vi "PH_Sequencer.ProcState.vi"(0 "i ref in":refnum<vi>, 2 "state timeout":i32=-1, 4 "state":string, 5 "error in (no error)":errorcluster) -> (14 "i ref out":refnum<vi>, 18 "next state":string, 19 "error out":errorcluster)   [LabVIEW 2014, in "PH_Sequencer.lvlib"]
doc: "This VI represents part of the internal state machine of the object. All methods that are needed to implement the required functionality of the state machine will be called from THIS VI. Add your code here."
uses:
  PH_Sequencer.lvlib
  PH_Beamline/PH_Beamline.Powermeter Instances.ctl
  Z6_Beamline/Z6_Beamline.Powermeter Instances.ctl
  PH_Basics/PH_PP_Common/PH_PP_Common.PUs.ctl
  CS_Core/CSSystem/CoreDefs/CoreDefs.error_type.ctl
  CS_Core/CSSystem/CoreLib/CoreLib.lvlib
  CS_Core/BaseSM/BaseSM.lvlib
  CS_Core/CSSystem/CSSystemLib/CSSystemLib.lvlib
  PH_Classes/PH_Calorimeter_USB/PH_Calorimeter_USB.lvlib
  PH_BackreflectionMeas/PH_BackreflectionMeas.lvlib
  PH_Basics/PH_Common/PH_Common.lvlib
  PH_Beamline/PH_Beamline.lvlib
  PH_Devices/PH_gentec_Powermeter/PH_gentec_Powermeter.lvlib
  Z6_Beamline/Z6_Beamline.lvlib
  PH_Devices/PH_Beckhoff_PPMA-Rods/PH_Beckhoff_PPMA-Rods.lvlib
  PH_BeamlineInformation/PH_BeamlineInformation.lvlib
  PH_Basics/PH_PP_Common/PH_PP_Common.lvlib
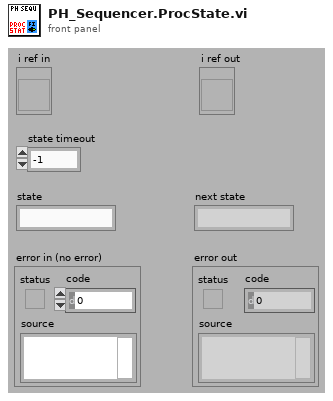
[diagram p1: front panel]
types:
  T1 = typedef "Z6_Beamline.lvlib/Z6_Beamline.Powermeter Instances.ctl" = string
  T2 = typedef "PH_Beamline.lvlib/PH_Beamline.Powermeter Instances.ctl" = string
  T3 = typedef "CoreDefs.error_type.ctl" = enum16{"no error", "can't load process", "can't unload process", "process does not exist", "can't install process", "can't remove process", "unknown function", "time out", "can't execute function", "duplicate queue name", "super not found", "caller queue invalid", "can't ping process", "unknown error", "VISA Error", "VISA timeout", "GPIB timeout", "GPIB error", "communication error", "data type mismatch", "can't read data from OPC server", "can't write data to OPC server", "OET error", "function not implemented", "process already exists", "invalid Shared Variable name", "error writing Shared Variable", "error reading Shared Variable", "invalid client name", "corrupt database", "unknown class", "call not authorized", "parameter out of range", "OET timeout: can't get data to modify", "invalid queue name", "requested operation incompatible with current state", "event undefined", "event disabled", "state undefined", "caller is not a friend", "EventBuilder: bad eventID", "EventBuilder: no DAQ devices", "a thread must not stop itself", "UNUSED ELEMENT4", "DiscArchiver: eventData incomplete", "DiscArchiver: eventData does not belong to run", "DiscArchiver: can't open file", "DiscArchiver: can't write to file", "DiscArchiver: available disc space low", "can't acquire semaphore", "error reading data from database", "notifier object is not existing", "can't register process", "can't unregister process", "illegal event type", "object disabled", "object already exists", "can't change state", "Instrument not found", "no connection to remote node", "invalid reference", "N/A", "UNUSED ELEMENT 1", "element not found", "illegal TCP/IP connection detected", "object does not exist", "invalid access ID", "unknown CS system", "invalid privilige", "unsupported data type", "unsupported server type", "IO server already exists", "Shared Variable already exists"}
  T4 = typedef "PH_Sequencer.lvlib/PH_Sequencer.i attribute.ctl" = cluster{"GUI Refs":cluster{"Main Off":refnum<vi>, "Fire":refnum<vi>, "Status":refnum<vi>, "Ready":refnum<vi>, "Waiting Time":refnum<vi>, "Timeout":refnum<vi>, "PPMA Ready":refnum<vi>, "Sequencer SM State":refnum<vi>, "PPPA Ready":refnum<vi>, "Calorimeter":refnum<vi>, "Beamline Ready":refnum<vi>, "Clear Beamline":refnum<vi>, "Linkage PPMA Rods":refnum<vi>, "Linkage Current PA":refnum<vi>, "Linkage Current MA":refnum<vi>, "Timing Ready":refnum<vi>, "State Timing":refnum<vi>, "Force Timing":refnum<vi>, "PSDB Shot Comment":refnum<vi>, "State PA Backreflection":refnum<vi>, "Beamline Z6 Ready":refnum<vi>, "Clear Z6 Beamline":refnum<vi>, "Sequence length":refnum<vi>, "Timing Mode":refnum<vi>, "Slow Trigger Settings":refnum<vi>, "Experiment Description":refnum<vi>, "State PSDB":refnum<vi>, "PSDB Ready":refnum<vi>, "Set PSDB Settings":refnum<vi>, "Get PSDB Info":refnum<vi>, "Take Snapshot":refnum<vi>, "Shottype":refnum<vi>, "Experiment":refnum<vi>, "Phase Frontends":refnum<vi>, "PP 45mm PILC in use":refnum<vi>}, "Status Info":cluster{"Machine Status":T5, "WaitingTime":i32, "Timeout":bool}, "Readyness":cluster{"Ready to shot":bool, "PPMA Ready":bool, "PPPA Ready":bool, "BL Ready":bool, "Timing Ready":bool, "BL Z6 Ready":bool, "PSDBReady":bool}, "Instancenames":cluster{"PPMA Rods":string, "PP Current Meas":string, "PH Beamline Chief":string, "PA Backrefl Meas":string, "Z6 Beamline Chief":string}, "Data to read":bool, "Calorimeter":cluster{"Instancename":string, "On":bool, "linked":bool}, "Linkage":cluster{"PPMA Rods":bool, "PP Current Meas":bool, "PHELIX Beamline Chief":bool, "PA Backrefl Meas":bool, "Z6 Beamline Chief":bool}, "Timing":cluster{"Instance":string, "linked":bool, "Status":T5, "Timing Mode":T6, "Slow Trigger Settings":T7, "Info available":cluster{"ext SlowTrigger":bool, "T2":bool, "Mode":bool, "Delay Slow Trigger":bool, "Phase FEs":bool}, "FE Phase":T8}, "Service ID R2S":i32, "PSDB":cluster{"Controller Instance":string, "Controller Status":T5, "Controller linked":bool, "Settings acknowledged":bool, "Current Experiment ID":i16, "Current Shot Type":i16, "Current Comment":string, "Remember Settings":bool, "Write 2 early":bool}, "PSDB Data":cluster{"Main Off?":bool, "Sequence Length":dbl, "Sequence startet":timestamp}, "6P 4Q Positions":cluster{"Instancename":string, "linked":bool, "Position":T9}[], "PUs":T10[]}
  T5 = typedef "PH_StatusHandler.lvlib/PH_StatusHandler.Status.ctl" = i16
  T6 = typedef "PH_Timing.lvlib/PH_Timing.Timing Mode.ctl" = cluster{"T2":i16, "Modeselector":enum32{"10 Hz", "0.5 Hz", "Shot"}}
  T7 = typedef "PH_Timing.lvlib/PH_Timing.Slow Trigger Settings.ctl" = cluster{"Delay":dbl, "externally triggered?":bool}
  T8 = typedef "PH_Timing.lvlib/PH_Timing.Phase FEs.ctl" = cluster{"Phase":dbl}
  T9 = typedef "PH_4_Pos_Selector.lvlib/PH_4_Pos_Selector.Position Selector.ctl" = u16
  T10 = typedef "PH_Sequencer.lvlib/PH_Sequencer.Head.ctl" = cluster{"PowerUnit":T11, "GUI Ref":refnum<vi>, "Information":T12, "linked?":bool, "GUI Ref Current Voltage":refnum<vi>}
  T11 = typedef "PH_PP_Common.lvlib/PH_PP_Common.PUs.ctl" = enum16{"no Info", "PA-19mm-1", "PA-19mm-2", "PA-45mm-PILC", "PA-45mm-MAIN", "MA-PU-1", "MA-PU-2", "MA-PU-3", "MA-PU-4", "MA-PU-5", "MA-PU-6", "MA-FR", "MA-PILC", "PA-45mm-DP"}
  T12 = typedef "PH_Sequencer.lvlib/PH_Sequencer.PU Information.ctl" = cluster{"State":T5, "Waiting Time [s]":dbl, "PU State SM":T13, "PU Timeout SM":T13}
  T13 = typedef "PH_PowerUnit_BaseClass.lvlib/PH_PowerUnit_BaseClass.SM States.ctl" = enum16{".", "Stand by", "Switch PU on", "Configure", "Set Default Voltage", "Set STANDBY", "Set READY", "Wait for Shot Cmd", "Open Dump Rods", "Open Ross Relais", "Close Ross Relais", "Switch PSU on", "Switch PSU off", "Charge", "Switch GD Channel on", "Close Dump Rods", "Rods-TO", "RR-TO", "PSU-TO", "Trigger-TO"}
  T14 = typedef "PH_BeamlineInformation.lvlib/PH_BeamlineInformation.i attribute.ctl" = cluster{"BL GUI Elements of Services":cluster{"Service Name":string, "GUI Elements":refnum<vi>[], "Status":i32}[], "Powermeters":T15, "Efficiency":T16, "Heads":T17[]}
  T15 = typedef "PH_BeamlineInformation.lvlib/PH_BeamlineInformation.Powermeter.ctl" = cluster{"ns FE":cluster{"GUI Ref":refnum<vi>, "Value":dbl}, "fs FE":cluster{"GUI Ref":refnum<vi>, "Value":dbl}, "PA":cluster{"GUI Ref":refnum<vi>, "Value":dbl}, "MA":cluster{"GUI Ref":refnum<vi>, "Value":dbl}, "Z6 green":cluster{"GUI Ref":refnum<vi>, "Value":dbl}, "Z6 IR":cluster{"GUI Ref":refnum<vi>, "Value":dbl}, "Z6 COS":cluster{"GUI Ref":refnum<vi>, "Value":dbl}}
  T16 = typedef "PH_BeamlineInformation.lvlib/PH_BeamlineInformation.Efficiency.ctl" = cluster{"PA Gain":cluster{"GUI Ref":refnum<vi>, "Value":dbl}, "MA Gain":cluster{"GUI Ref":refnum<vi>, "Value":dbl}, "Z6 green Conversion":cluster{"GUI Ref":refnum<vi>, "Value":dbl}, "Z6 Comp Losses":cluster{"GUI Ref":refnum<vi>, "Value":dbl}}
  T17 = typedef "PH_BeamlineInformation.lvlib/PH_BeamlineInformation.Head.ctl" = cluster{"PowerUnit":T11, "in use":cluster{"Value":bool, "GUI Ref":refnum<vi>, "linked":bool}, "voltage":cluster{"Value":dbl, "GUI Ref":refnum<vi>, "linked":bool}}
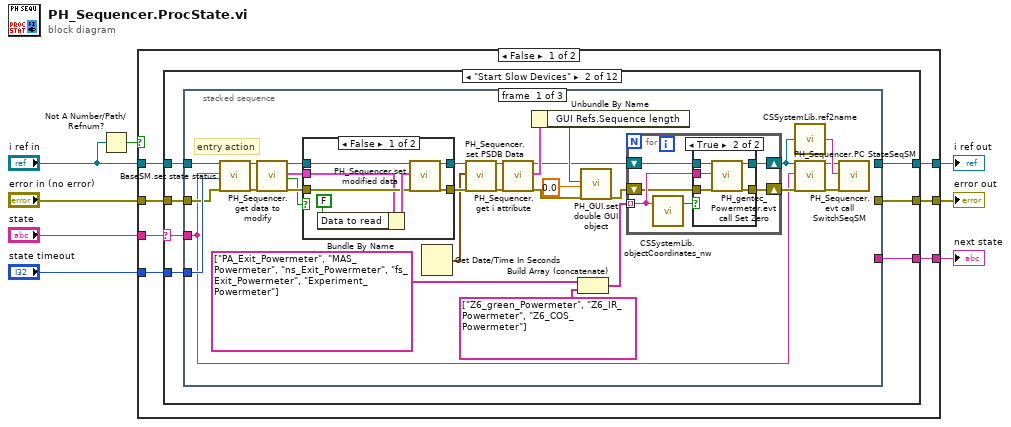
[diagram p0: block diagram]
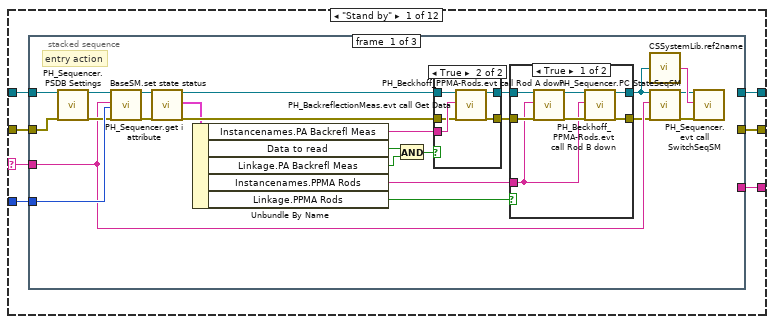
[diagram p2: hidden frame]
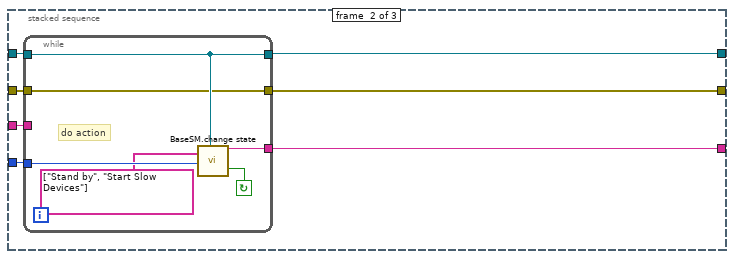
[diagram p5: hidden frame]
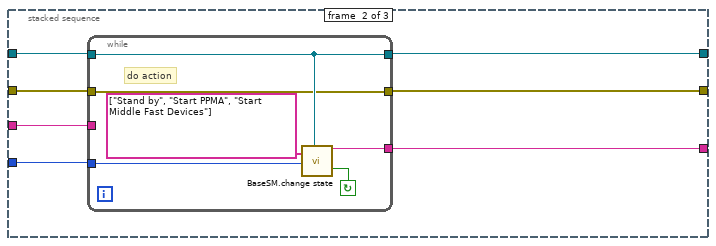
[diagram p9: hidden frame]
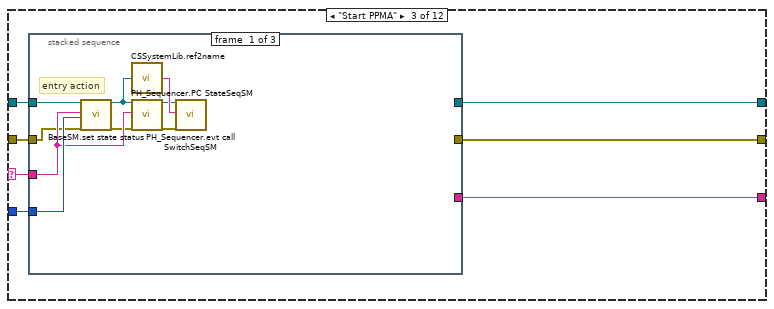
[diagram p11: hidden frame]
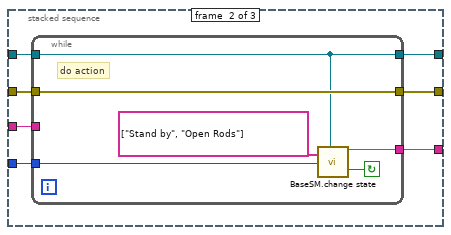
[diagram p12: hidden frame]
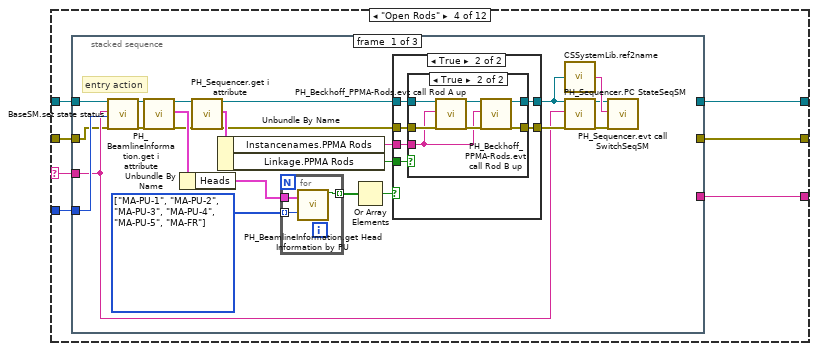
[diagram p14: hidden frame]
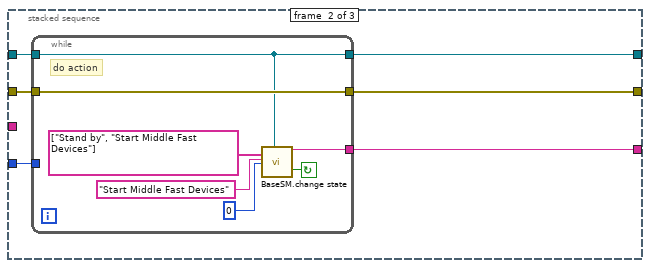
[diagram p17: hidden frame]
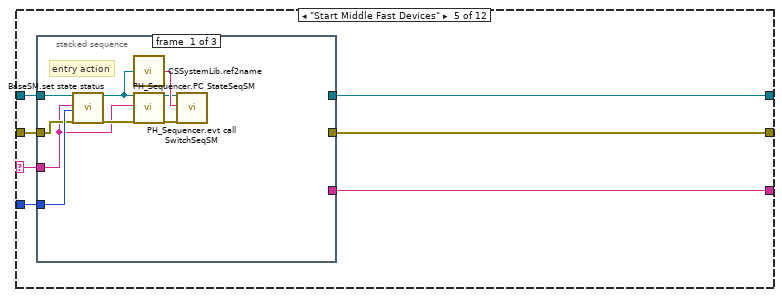
[diagram p19: hidden frame]
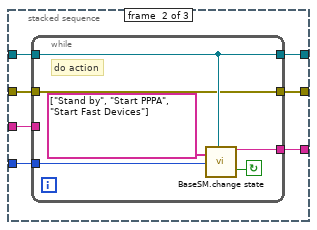
[diagram p20: hidden frame]
diagram:
  n1 = Not A Number/Path/Refnum?(number/path/refnum="i ref in") -> (NaN/Path/Refnum?=w2:bool)
  n2 = case shown="False" w2 {
    tunnel: "i ref in" -> [w15 w474]
    tunnel: [w14 w474] -> w8
    tunnel: "state" -> [w13 w471]
    tunnel: [w12 w471] -> w6
    tunnel: "state timeout" -> [w11 _]
    tunnel: "error in (no error)" -> [w10 _]
    tunnel: [w9 w472] -> w3
    frame False {
      n3 = case shown="\"Start Slow Devices\"" w13 {
        selector: w13 -> [w22 w82 w153 w181 w242 w271 w301 w344 w372 w400 w428 w465]
        tunnel: w15 -> [w20 w80 w151 w179 w240 w269 w299 w342 w370 w398 w426 w470]
        tunnel: [w19 w79 w150 w178 w239 w268 w298 w341 w369 w397 w425 w469] -> w14
        tunnel: [w21 w81 w152 w180 w241 w270 w300 w343 w371 w399 w427 w464] -> w12
        tunnel: w11 -> [w18 w78 w149 w177 w238 w267 w297 w340 w368 w396 w424 w466]
        tunnel: w10 -> [w17 w77 w148 w176 w237 w266 w296 w339 w367 w395 w423 w468]
        tunnel: [w16 w76 w147 w175 w236 w265 w295 w338 w366 w394 w422 w467] -> w9
        frame "Stand by" {
          n4 = stacked-sequence {
            tunnel: w22 -> [w31 w69 _]
            tunnel: [_ w68 _] -> w21
            tunnel: w20 -> [w40 w66 _]
            tunnel: [_ w65 _] -> w19
            tunnel: w18 -> [w39 w67 _]
            tunnel: w17 -> [w42 w63 _]
            tunnel: [_ w64 _] -> w16
            frame #0 {
              # "entry action"
              n5 = call "PH_Sequencer.PSDB Settings.vi"("i ref in"=w40, "error in"=w42) -> ("i ref out"=w38:refnum<vi>, "error out"=w36:errorcluster)  [unwired: 16 in]
              n6 = call "BaseSM.set state status.vi"("i ref in"=w38, "stateStatus"=w31, "ms timeout (10000)"=w39, "error in (no error)"=w36) -> ("i ref out"=w37:refnum<vi>, "error out"=w35:errorcluster)  [unwired: 13 in, 1 out]
              n7 = call "PH_Sequencer.get i attribute.vi"("i ref in"=w37, "error in (no error)"=w35) -> ("i ref out"=w44:refnum<vi>, "i attribute"=w41:T4, "error out"=w43:errorcluster)  [unwired: 15 in]
              n8 = Unbundle By Name(w41) -> ("Instancenames.PA Backrefl Meas"=w23:string, "Data to read"=w25:bool, "Linkage.PA Backrefl Meas"=w24:bool, "Instancenames.PPMA Rods"=w30:string, "Linkage.PPMA Rods"=w29:bool)
              n9 = And(x=w25, y=w24) -> (x .and. y?=w26:bool)
              n10 = case shown="True" w26 {
                tunnel: w44 -> [w48 w49]
                tunnel: [w48 w53] -> w46
                tunnel: w43 -> [w47 w50]
                tunnel: [w47 w52] -> w45
                tunnel: w23 -> [_ w51]
                frame False {
                }
                frame True {
                  n11 = call "PH_BackreflectionMeas.evt call Get Data.vi"("i ref in"=w49, "Instance"=w51, "error in (no error)"=w50) -> ("i ref out"=w53:refnum<vi>, "error out"=w52:errorcluster)  [unwired: 15 in]
                }
              }
              n12 = case shown="True" w29 {
                tunnel: w46 -> [w60 w62]
                tunnel: [w55 w62] -> w28
                tunnel: w45 -> [w59 w61]
                tunnel: [w57 w61] -> w27
                tunnel: w30 -> [w54 _]
                frame True {
                  n13 = call "PH_Beckhoff_PPMA-Rods.evt call Rod A down.vi"("i ref in"=w60, "Instance name"=w54, "error in"=w59) -> ("i ref out"=w56:refnum<vi>, "error out"=w58:errorcluster)  [unwired: 15 in]
                  n14 = call "PH_Beckhoff_PPMA-Rods.evt call Rod B down.vi"("i ref in"=w56, "Instance name"=w54, "error in"=w58) -> ("i ref out"=w55:refnum<vi>, "error out"=w57:errorcluster)  [unwired: 15 in]
                }
                frame False {
                }
              }
              n15 = call "CSSystemLib.ref2name.vi"("obj refnum"=w28) -> ("name"=w34:string)
              n16 = call "PH_Sequencer.PC StateSeqSM.vi"("i ref in"=w28, "Seq SM State"=w31, "error in (no error)"=w27) -> ("i ref out"=w33:refnum<vi>, "error out"=w32:errorcluster)  [unwired: 15 in]
              n17 = call "PH_Sequencer.evt call SwitchSeqSM.vi"("i ref in"=w33, "Instance"=w34, "error in (no error)"=w32) -> ()  [unwired: 15 in, 2 out]
            }
            frame #1 {
              n18 = while {
                tunnel: w67 -> [w73]
                tunnel: [w75] -> w68
                tunnel: w69 -> [_]
                tunnel: w66 -> [w72]
                tunnel: [w72] -> w65
                tunnel: [w71] -> w64
                tunnel: w63 -> [w71]
                stop <- w74 continue-if-true
                # "do action"
                n19 = call "BaseSM.change state.vi"("allowed next states"=string[] ["Stand by", "Start Slow Devices"], "wait time [ms]"=w73, "i ref in"=w72) -> ("next state"=w75:string, "continue loop"=w74:bool)  [unwired: 13 in, 2 out]
              }
            }
            frame #2 {
              # "exit action"
            }
          }
        }
        frame "Start Slow Devices" {
          n20 = stacked-sequence {
            tunnel: w82 -> [w87 w140 _]
            tunnel: [_ w139 _] -> w81
            tunnel: w80 -> [w110 w137 _]
            tunnel: [_ w136 _] -> w79
            tunnel: w78 -> [w111 w138 _]
            tunnel: w77 -> [w109 w134 _]
            tunnel: [_ w135 _] -> w76
            frame #0 {
              # "entry action"
              n21 = call "BaseSM.set state status.vi"("i ref in"=w110, "stateStatus"=w87, "ms timeout (10000)"=w111, "error in (no error)"=w109) -> ("i ref out"=w108:refnum<vi>, "error out"=w106:errorcluster)  [unwired: 13 in, 1 out]
              n22 = call "PH_Sequencer.get data to modify.vi"("i ref in"=w108, "error in (no error)"=w106) -> ("i ref out"=w107:refnum<vi>, "i attribute"=w103:T4, "timed out"=w104:bool, "error out"=w105:errorcluster)  [unwired: 14 in]
              n23 = case shown="False" w104 {
                tunnel: w103 -> [w127 _]
                tunnel: w107 -> [w129 w133]
                tunnel: w105 -> [w128 w132]
                tunnel: [w126 w133] -> w94
                tunnel: [w125 w132] -> w96
                frame False {
                  n24 = Bundle By Name(cluster=w127, "Data to read"=FALSE) -> (w131:T4)
                  n25 = call "PH_Sequencer.set modified data.vi"("i ref in"=w129, "i attribute"=w131, "error in (no error)"=w128) -> ("i ref out"=w126:refnum<vi>, "error out"=w125:errorcluster)  [unwired: 15 in]
                }
                frame True {
                }
              }
              n26 = Get Date/Time In Seconds() -> (seconds since 1Jan1904=w93:timestamp)
              n27 = call "PH_Sequencer.set PSDB Data.vi"("i ref in"=w94, "Start Sequence Time (0)"=w93, "error in"=w96) -> ("i ref out"=w95:refnum<vi>, "error out"=w97:errorcluster)  [unwired: 15 in]
              n28 = call "PH_Sequencer.get i attribute.vi"("i ref in"=w95, "error in (no error)"=w97) -> ("i ref out"=w84:refnum<vi>, "i attribute"=w102:T4, "error out"=w83:errorcluster)  [unwired: 15 in]
              n29 = Unbundle By Name(w102) -> ("GUI Refs.Sequence length"=w101:refnum<vi>)
              n30 = Build Array (concatenate)(T2[] ["PA_Exit_Powermeter", "MAS_Powermeter", "ns_Exit_Powermeter", "fs_Exit_Powermeter", "Experiment_Powermeter"], T1[] ["Z6_green_Powermeter", "Z6_IR_Powermeter", "Z6_COS_Powermeter"]) -> (w98:T1[])
              n31 = call "PH_GUI.set double GUI object.vi"("GUI object Ref"=w101, "value"=0.0, "error in (no error)"=w83) -> ("error out"=w86:errorcluster)  [unwired: 16 in]
              n32 = for {
                tunnel: w98 -> [w117] mode=indexing
                shift-right: [w115] -> w89
                shift-left: w84 -> [w114]
                shift-right: [w113] -> w88
                shift-left: w86 -> [w112]
                n33 = call "CSSystemLib.objectCoordinates_nw.vi"("name"=w117) -> ("obj exists"=w116:bool)  [unwired: 15 in, 3 out]
                n34 = case shown="True" w116 {
                  tunnel: w117 -> [_ w124]
                  tunnel: [w119 w123] -> w115
                  tunnel: w114 -> [w119 w122]
                  tunnel: [w118 w121] -> w113
                  tunnel: w112 -> [w118 w120]
                  frame False {
                  }
                  frame True {
                    n35 = call "PH_gentec_Powermeter.evt call Set Zero.vi"("i ref in"=w122, "Instance"=w124, "error in (no error)"=w120) -> ("i ref out"=w123:refnum<vi>, "error out"=w121:errorcluster)  [unwired: 15 in]
                  }
                }
              }
              n36 = call "CSSystemLib.ref2name.vi"("obj refnum"=w89) -> ("name"=w92:string)
              n37 = call "PH_Sequencer.PC StateSeqSM.vi"("i ref in"=w89, "Seq SM State"=w87, "error in (no error)"=w88) -> ("i ref out"=w91:refnum<vi>, "error out"=w90:errorcluster)  [unwired: 15 in]
              n38 = call "PH_Sequencer.evt call SwitchSeqSM.vi"("i ref in"=w91, "Instance"=w92, "error in (no error)"=w90) -> ()  [unwired: 15 in, 2 out]
            }
            frame #1 {
              n39 = while {
                tunnel: w138 -> [w141]
                tunnel: [w146] -> w139
                tunnel: w140 -> [_]
                tunnel: w137 -> [w144]
                tunnel: [w144] -> w136
                tunnel: [w143] -> w135
                tunnel: w134 -> [w143]
                stop <- w145 continue-if-true
                # "do action"
                n40 = call "BaseSM.change state.vi"("allowed next states"=string[] ["Stand by", "Start PPMA", "Start Middle Fast Devices"], "wait time [ms]"=w141, "i ref in"=w144) -> ("next state"=w146:string, "continue loop"=w145:bool)  [unwired: 13 in, 2 out]
              }
            }
            frame #2 {
              # "exit action"
            }
          }
        }
        frame "Start PPMA" {
          n41 = stacked-sequence {
            tunnel: w153 -> [w158 w168 _]
            tunnel: [_ w167 _] -> w152
            tunnel: w151 -> [w160 w165 _]
            tunnel: [_ w164 _] -> w150
            tunnel: w149 -> [w161 w166 _]
            tunnel: w148 -> [w155 w162 _]
            tunnel: [_ w163 _] -> w147
            frame #0 {
              # "entry action"
              n42 = call "BaseSM.set state status.vi"("i ref in"=w160, "stateStatus"=w158, "ms timeout (10000)"=w161, "error in (no error)"=w155) -> ("i ref out"=w154:refnum<vi>)  [unwired: 13 in, 2 out]
              n43 = call "CSSystemLib.ref2name.vi"("obj refnum"=w154) -> ("name"=w159:string)
              n44 = call "PH_Sequencer.PC StateSeqSM.vi"("i ref in"=w154, "Seq SM State"=w158, "error in (no error)"=w155) -> ("i ref out"=w157:refnum<vi>, "error out"=w156:errorcluster)  [unwired: 15 in]
              n45 = call "PH_Sequencer.evt call SwitchSeqSM.vi"("i ref in"=w157, "Instance"=w159, "error in (no error)"=w156) -> ()  [unwired: 15 in, 2 out]
            }
            frame #1 {
              n46 = while {
                tunnel: w166 -> [w171]
                tunnel: [w174] -> w167
                tunnel: w168 -> [_]
                tunnel: w165 -> [w169]
                tunnel: [w169] -> w164
                tunnel: [w170] -> w163
                tunnel: w162 -> [w170]
                stop <- w173 continue-if-true
                # "do action"
                n47 = call "BaseSM.change state.vi"("allowed next states"=string[] ["Stand by", "Open Rods"], "wait time [ms]"=w171, "i ref in"=w169) -> ("next state"=w174:string, "continue loop"=w173:bool)  [unwired: 13 in, 2 out]
              }
            }
            frame #2 {
              # "exit action"
            }
          }
        }
        frame "Open Rods" {
          n48 = stacked-sequence {
            tunnel: w181 -> [w198 _ _]
            tunnel: [_ w228 _] -> w180
            tunnel: w179 -> [w188 w226 _]
            tunnel: [_ w225 _] -> w178
            tunnel: w177 -> [w202 w227 _]
            tunnel: w176 -> [w186 w223 _]
            tunnel: [_ w224 _] -> w175
            frame #0 {
              w182 = T11[] [enum."MA-PU-1", enum."MA-PU-2", enum."MA-PU-3", enum."MA-PU-4", enum."MA-PU-5", enum."MA-FR"] items=["no Info", "PA-19mm-1", "PA-19mm-2", "PA-45mm-PILC", "PA-45mm-MAIN", "MA-PU-1", "MA-PU-2", "MA-PU-3", "MA-PU-4", "MA-PU-5", "MA-PU-6", "MA-FR", "MA-PILC", "PA-45mm-DP"]
              # "entry action"
              n49 = call "BaseSM.set state status.vi"("i ref in"=w188, "stateStatus"=w198, "ms timeout (10000)"=w202, "error in (no error)"=w186) -> ()  [unwired: 13 in, 3 out]
              n50 = call "PH_BeamlineInformation.get i attribute.vi"("i ref in"=w188, "error in (no error)"=w186) -> ("i ref out"=w187:refnum<vi>, "i attribute"=w189:T14, "error out"=w185:errorcluster)  [unwired: 15 in]
              n51 = Unbundle By Name(w189) -> ("Heads"=w184:T17[])
              n52 = call "PH_Sequencer.get i attribute.vi"("i ref in"=w187, "error in (no error)"=w185) -> ("i ref out"=w193:refnum<vi>, "i attribute"=w197:T4, "error out"=w194:errorcluster)  [unwired: 15 in]
              n53 = Unbundle By Name(w197) -> ("Instancenames.PPMA Rods"=w196:string, "Linkage.PPMA Rods"=w195:bool)
              n54 = for {
                tunnel: [w205] -> w183 mode=indexing
                tunnel: w184 -> [w204]
                tunnel: w182 -> [w203] mode=indexing
                n55 = call "PH_BeamlineInformation.get Head Information by PU.vi"("Heads"=w204, "Power Unit"=w203) -> ("In Use?"=w205:bool)  [unwired: 12 in, 5 out]
              }
              n56 = Or Array Elements(Boolean array=w183) -> (logical OR=w201:bool)
              n57 = case shown="True" w201 {
                tunnel: w193 -> [w207 w213]
                tunnel: [w207 w212] -> w190
                tunnel: w194 -> [w206 w211]
                tunnel: [w206 w210] -> w199
                tunnel: w196 -> [_ w209]
                tunnel: w195 -> [_ w208]
                frame False {
                }
                frame True {
                  n58 = case shown="True" w208 {
                    tunnel: w213 -> [w215 w222]
                    tunnel: [w215 w216] -> w212
                    tunnel: w211 -> [w214 w221]
                    tunnel: [w214 w219] -> w210
                    tunnel: w209 -> [_ w218]
                    frame False {
                    }
                    frame True {
                      n59 = call "PH_Beckhoff_PPMA-Rods.evt call Rod A up.vi"("i ref in"=w222, "Instance name"=w218, "error in"=w221) -> ("i ref out"=w217:refnum<vi>, "error out"=w220:errorcluster)  [unwired: 15 in]
                      n60 = call "PH_Beckhoff_PPMA-Rods.evt call Rod B up.vi"("i ref in"=w217, "Instance name"=w218, "error in"=w220) -> ("i ref out"=w216:refnum<vi>, "error out"=w219:errorcluster)  [unwired: 15 in]
                    }
                  }
                }
              }
              n61 = call "CSSystemLib.ref2name.vi"("obj refnum"=w190) -> ("name"=w200:string)
              n62 = call "PH_Sequencer.PC StateSeqSM.vi"("i ref in"=w190, "Seq SM State"=w198, "error in (no error)"=w199) -> ("i ref out"=w191:refnum<vi>, "error out"=w192:errorcluster)  [unwired: 15 in]
              n63 = call "PH_Sequencer.evt call SwitchSeqSM.vi"("i ref in"=w191, "Instance"=w200, "error in (no error)"=w192) -> ()  [unwired: 15 in, 2 out]
            }
            frame #1 {
              n64 = while {
                tunnel: w227 -> [_]
                tunnel: [w235] -> w228
                tunnel: w226 -> [w229]
                tunnel: [w229] -> w225
                tunnel: [w230] -> w224
                tunnel: w223 -> [w230]
                stop <- w234 continue-if-true
                # "do action"
                n65 = call "BaseSM.change state.vi"("allowed next states"=string[] ["Stand by", "Start Middle Fast Devices"], "default state"="Start Middle Fast Devices", "wait time [ms]"=0 ("wait time"), "i ref in"=w229) -> ("next state"=w235:string, "continue loop"=w234:bool)  [unwired: 12 in, 2 out]
              }
            }
            frame #2 {
              # "exit action"
            }
          }
        }
        frame "Start Middle Fast Devices" {
          n66 = stacked-sequence {
            tunnel: w242 -> [w246 w258 _]
            tunnel: [_ w257 _] -> w241
            tunnel: w240 -> [w250 w255 _]
            tunnel: [_ w254 _] -> w239
            tunnel: w238 -> [w251 w256 _]
            tunnel: w237 -> [w249 w252 _]
            tunnel: [_ w253 _] -> w236
            frame #0 {
              # "entry action"
              n67 = call "BaseSM.set state status.vi"("i ref in"=w250, "stateStatus"=w246, "ms timeout (10000)"=w251, "error in (no error)"=w249) -> ("i ref out"=w244:refnum<vi>, "error out"=w247:errorcluster)  [unwired: 13 in, 1 out]
              n68 = call "CSSystemLib.ref2name.vi"("obj refnum"=w244) -> ("name"=w248:string)
              n69 = call "PH_Sequencer.PC StateSeqSM.vi"("i ref in"=w244, "Seq SM State"=w246, "error in (no error)"=w247) -> ("i ref out"=w243:refnum<vi>, "error out"=w245:errorcluster)  [unwired: 15 in]
              n70 = call "PH_Sequencer.evt call SwitchSeqSM.vi"("i ref in"=w243, "Instance"=w248, "error in (no error)"=w245) -> ()  [unwired: 15 in, 2 out]
            }
            frame #1 {
              n71 = while {
                tunnel: w256 -> [w259]
                tunnel: [w264] -> w257
                tunnel: w258 -> [_]
                tunnel: w255 -> [w262]
                tunnel: [w262] -> w254
                tunnel: [w261] -> w253
                tunnel: w252 -> [w261]
                stop <- w263 continue-if-true
                # "do action"
                n72 = call "BaseSM.change state.vi"("allowed next states"=string[] ["Stand by", "Start PPPA", "Start Fast Devices"], "wait time [ms]"=w259, "i ref in"=w262) -> ("next state"=w264:string, "continue loop"=w263:bool)  [unwired: 13 in, 2 out]
              }
            }
            frame #2 {
              # "exit action"
            }
          }
        }
        frame "Start PPPA" {
          # "To wait for 2.5 s is due to PA 45mm DP:\nWithin this state, the hardware gets ready (takes some time)\nat \"Start Fast Devices\" the charge command is given."
          n73 = stacked-sequence {
            tunnel: w271 -> [w278 w287 _]
            tunnel: [_ w286 _] -> w270
            tunnel: w269 -> [w275 w284 _]
            tunnel: [_ w283 _] -> w268
            tunnel: w267 -> [w280 w285 _]
            tunnel: w266 -> [w274 w281 _]
            tunnel: [_ w282 _] -> w265
            frame #0 {
              # "entry action"
              n74 = call "BaseSM.set state status.vi"("i ref in"=w275, "stateStatus"=w278, "ms timeout (10000)"=w280, "error in (no error)"=w274) -> ("i ref out"=w273:refnum<vi>, "error out"=w272:errorcluster)  [unwired: 13 in, 1 out]
              n75 = call "CSSystemLib.ref2name.vi"("obj refnum"=w273) -> ("name"=w279:string)
              n76 = call "PH_Sequencer.PC StateSeqSM.vi"("i ref in"=w273, "Seq SM State"=w278, "error in (no error)"=w272) -> ("i ref out"=w276:refnum<vi>, "error out"=w277:errorcluster)  [unwired: 15 in]
              n77 = call "PH_Sequencer.evt call SwitchSeqSM.vi"("i ref in"=w276, "Instance"=w279, "error in (no error)"=w277) -> ()  [unwired: 15 in, 2 out]
            }
            frame #1 {
              n78 = while {
                tunnel: w285 -> [_]
                tunnel: [w294] -> w286
                tunnel: w287 -> [_]
                tunnel: w284 -> [w288]
                tunnel: [w288] -> w283
                tunnel: [w289] -> w282
                tunnel: w281 -> [w289]
                stop <- w293 continue-if-true
                # "do action"
                n79 = call "BaseSM.change state.vi"("allowed next states"=string[] ["Stand by", "Start Fast Devices"], "default state"="Start Fast Devices", "wait time [ms]"=2500 ("wait time"), "i ref in"=w288) -> ("next state"=w294:string, "continue loop"=w293:bool)  [unwired: 12 in, 2 out]
              }
            }
            frame #2 {
              # "exit action"
            }
          }
        }
        frame "Start Fast Devices" {
          n80 = stacked-sequence {
            tunnel: w301 -> [w315 w331 _]
            tunnel: [_ w330 _] -> w300
            tunnel: w299 -> [w303 w328 _]
            tunnel: [_ w327 _] -> w298
            tunnel: w297 -> [w317 w329 _]
            tunnel: w296 -> [w302 w325 _]
            tunnel: [_ w326 _] -> w295
            frame #0 {
              # "entry action"
              n81 = call "BaseSM.set state status.vi"("i ref in"=w303, "stateStatus"=w315, "ms timeout (10000)"=w317, "error in (no error)"=w302) -> ()  [unwired: 13 in, 3 out]
              n82 = call "PH_Sequencer.get i attribute.vi"("i ref in"=w303, "error in (no error)"=w302) -> ("i ref out"=w309:refnum<vi>, "i attribute"=w314:T4, "error out"=w308:errorcluster)  [unwired: 15 in]
              n83 = Unbundle By Name(w314) -> ("Calorimeter.Instancename"=w311:string, "Calorimeter.On"=w313:bool, "Calorimeter.linked"=w310:bool)
              n84 = And(x=w313, y=w310) -> (x .and. y?=w312:bool)
              n85 = case shown="True" w312 {
                tunnel: [w318 w324] -> w307
                tunnel: [w319 w323] -> w304
                tunnel: w308 -> [w318 w322]
                tunnel: w309 -> [w319 w321]
                tunnel: w311 -> [_ w320]
                frame False {
                }
                frame True {
                  n86 = call "PH_Calorimeter_USB.evt call Start.vi"("i ref in"=w321, "Calorimeter Instance"=w320, "error in (no error)"=w322) -> ("i ref out"=w323:refnum<vi>, "error out"=w324:errorcluster)  [unwired: 15 in]
                }
              }
              n87 = call "PH_Sequencer.PC StateSeqSM.vi"("i ref in"=w304, "Seq SM State"=w315, "error in (no error)"=w307) -> ("i ref out"=w305:refnum<vi>, "error out"=w306:errorcluster)  [unwired: 15 in]
              n88 = call "CSSystemLib.ref2name.vi"("obj refnum"=w304) -> ("name"=w316:string)
              n89 = call "PH_Sequencer.evt call SwitchSeqSM.vi"("i ref in"=w305, "Instance"=w316, "error in (no error)"=w306) -> ()  [unwired: 15 in, 2 out]
            }
            frame #1 {
              n90 = while {
                tunnel: w329 -> [_]
                tunnel: [w337] -> w330
                tunnel: w331 -> [_]
                tunnel: w328 -> [w334]
                tunnel: [w334] -> w327
                tunnel: [w333] -> w326
                tunnel: w325 -> [w333]
                stop <- w336 continue-if-true
                # "do action"
                n91 = call "BaseSM.change state.vi"("allowed next states"=string[] ["Stand by", "Enable Sub-GDs"], "wait time [ms]"=1000, "i ref in"=w334) -> ("next state"=w337:string, "continue loop"=w336:bool)  [unwired: 13 in, 2 out]
              }
            }
            frame #2 {
              # "exit action"
            }
          }
        }
        frame "Enable Sub-GDs" {
          n92 = stacked-sequence {
            tunnel: w344 -> [w349 w358 _]
            tunnel: [_ w357 _] -> w343
            tunnel: w342 -> [w347 w355 _]
            tunnel: [_ w354 _] -> w341
            tunnel: w340 -> [w351 w356 _]
            tunnel: w339 -> [w348 w352 _]
            tunnel: [_ w353 _] -> w338
            frame #0 {
              # "entry action"
              n93 = call "BaseSM.set state status.vi"("i ref in"=w347, "stateStatus"=w349, "ms timeout (10000)"=w351, "error in (no error)"=w348) -> ()  [unwired: 13 in, 3 out]
              n94 = call "CSSystemLib.ref2name.vi"("obj refnum"=w347) -> ("name"=w350:string)
              n95 = call "PH_Sequencer.PC StateSeqSM.vi"("i ref in"=w347, "Seq SM State"=w349, "error in (no error)"=w348) -> ("i ref out"=w346:refnum<vi>, "error out"=w345:errorcluster)  [unwired: 15 in]
              n96 = call "PH_Sequencer.evt call SwitchSeqSM.vi"("i ref in"=w346, "Instance"=w350, "error in (no error)"=w345) -> ()  [unwired: 15 in, 2 out]
            }
            frame #1 {
              n97 = while {
                tunnel: w356 -> [_]
                tunnel: [w365] -> w357
                tunnel: w358 -> [_]
                tunnel: w355 -> [w363]
                tunnel: [w363] -> w354
                tunnel: [w362] -> w353
                tunnel: w352 -> [w362]
                stop <- w364 continue-if-true
                # "do action"
                n98 = call "BaseSM.change state.vi"("allowed next states"=string[] ["Stand by", "Enable Master-GD Channels"], "default state"="Enable Master-GD Channels", "wait time [ms]"=1000 ("state timeout"), "i ref in"=w363) -> ("next state"=w365:string, "continue loop"=w364:bool)  [unwired: 12 in, 2 out]
              }
            }
            frame #2 {
              # "exit action"
            }
          }
        }
        frame "Enable Master-GD Channels" {
          n99 = stacked-sequence {
            tunnel: w372 -> [w377 w386 _]
            tunnel: [_ w385 _] -> w371
            tunnel: w370 -> [w376 w383 _]
            tunnel: [_ w382 _] -> w369
            tunnel: w368 -> [w379 w384 _]
            tunnel: w367 -> [w375 w380 _]
            tunnel: [_ w381 _] -> w366
            frame #0 {
              # "entry action"
              n100 = call "BaseSM.set state status.vi"("i ref in"=w376, "stateStatus"=w377, "ms timeout (10000)"=w379, "error in (no error)"=w375) -> ()  [unwired: 13 in, 3 out]
              n101 = call "CSSystemLib.ref2name.vi"("obj refnum"=w376) -> ("name"=w378:string)
              n102 = call "PH_Sequencer.PC StateSeqSM.vi"("i ref in"=w376, "Seq SM State"=w377, "error in (no error)"=w375) -> ("i ref out"=w374:refnum<vi>, "error out"=w373:errorcluster)  [unwired: 15 in]
              n103 = call "PH_Sequencer.evt call SwitchSeqSM.vi"("i ref in"=w374, "Instance"=w378, "error in (no error)"=w373) -> ()  [unwired: 15 in, 2 out]
            }
            frame #1 {
              n104 = while {
                tunnel: w384 -> [_]
                tunnel: [w393] -> w385
                tunnel: w386 -> [_]
                tunnel: w383 -> [w391]
                tunnel: [w391] -> w382
                tunnel: [w390] -> w381
                tunnel: w380 -> [w390]
                stop <- w392 continue-if-true
                # "do action"
                n105 = call "BaseSM.change state.vi"("allowed next states"=string[] ["Stand by", "Enable Master-GD"], "default state"="Enable Master-GD", "wait time [ms]"=1000 ("state timeout"), "i ref in"=w391) -> ("next state"=w393:string, "continue loop"=w392:bool)  [unwired: 12 in, 2 out]
              }
            }
            frame #2 {
              # "exit action"
            }
          }
        }
        frame "Enable Master-GD" {
          n106 = stacked-sequence {
            tunnel: w400 -> [w405 w414 _]
            tunnel: [_ w413 _] -> w399
            tunnel: w398 -> [w402 w411 _]
            tunnel: [_ w410 _] -> w397
            tunnel: w396 -> [w407 w412 _]
            tunnel: w395 -> [w404 w408 _]
            tunnel: [_ w409 _] -> w394
            frame #0 {
              # "entry action"
              n107 = call "BaseSM.set state status.vi"("i ref in"=w402, "stateStatus"=w405, "ms timeout (10000)"=w407, "error in (no error)"=w404) -> ()  [unwired: 13 in, 3 out]
              n108 = call "CSSystemLib.ref2name.vi"("obj refnum"=w402) -> ("name"=w406:string)
              n109 = call "PH_Sequencer.PC StateSeqSM.vi"("i ref in"=w402, "Seq SM State"=w405, "error in (no error)"=w404) -> ("i ref out"=w401:refnum<vi>, "error out"=w403:errorcluster)  [unwired: 15 in]
              n110 = call "PH_Sequencer.evt call SwitchSeqSM.vi"("i ref in"=w401, "Instance"=w406, "error in (no error)"=w403) -> ()  [unwired: 15 in, 2 out]
            }
            frame #1 {
              n111 = while {
                tunnel: w412 -> [_]
                tunnel: [w421] -> w413
                tunnel: w414 -> [_]
                tunnel: w411 -> [w419]
                tunnel: [w419] -> w410
                tunnel: [w418] -> w409
                tunnel: w408 -> [w418]
                stop <- w420 continue-if-true
                # "do action"
                n112 = call "BaseSM.change state.vi"("allowed next states"=string[] ["Stand by", "Enable Data Acquisition"], "default state"="Enable Data Acquisition", "wait time [ms]"=0 ("state timeout"), "i ref in"=w419) -> ("next state"=w421:string, "continue loop"=w420:bool)  [unwired: 12 in, 2 out]
              }
            }
            frame #2 {
              # "exit action"
            }
          }
        }
        frame "Enable Data Acquisition" {
          n113 = stacked-sequence {
            tunnel: w428 -> [w432 w457 _]
            tunnel: [_ w456 _] -> w427
            tunnel: w426 -> [w440 w454 _]
            tunnel: [_ w453 _] -> w425
            tunnel: w424 -> [w441 w455 _]
            tunnel: w423 -> [w439 w451 _]
            tunnel: [_ w452 _] -> w422
            frame #0 {
              # "entry action"
              n114 = call "BaseSM.set state status.vi"("i ref in"=w440, "stateStatus"=w432, "ms timeout (10000)"=w441, "error in (no error)"=w439) -> ()  [unwired: 13 in, 3 out]
              n115 = call "PH_Sequencer.get data to modify.vi"("i ref in"=w440, "error in (no error)"=w439) -> ("i ref out"=w437:refnum<vi>, "i attribute"=w438:T4, "timed out"=w435:bool, "error out"=w436:errorcluster)  [unwired: 14 in]
              n116 = case shown="False" w435 {
                tunnel: w438 -> [w446 _]
                tunnel: w437 -> [w448 w450]
                tunnel: w436 -> [w447 w449]
                tunnel: [w443 w449] -> w433
                tunnel: [w442 w450] -> w429
                frame False {
                  n117 = Bundle By Name(cluster=w446, "Data to read"=TRUE) -> (w445:T4)
                  n118 = call "PH_Sequencer.set modified data.vi"("i ref in"=w448, "i attribute"=w445, "error in (no error)"=w447) -> ("i ref out"=w442:refnum<vi>, "error out"=w443:errorcluster)  [unwired: 15 in]
                }
                frame True {
                }
              }
              n119 = call "CSSystemLib.ref2name.vi"("obj refnum"=w429) -> ("name"=w434:string)
              n120 = call "PH_Sequencer.PC StateSeqSM.vi"("i ref in"=w429, "Seq SM State"=w432, "error in (no error)"=w433) -> ("i ref out"=w430:refnum<vi>, "error out"=w431:errorcluster)  [unwired: 15 in]
              n121 = call "PH_Sequencer.evt call SwitchSeqSM.vi"("i ref in"=w430, "Instance"=w434, "error in (no error)"=w431) -> ()  [unwired: 15 in, 2 out]
            }
            frame #1 {
              n122 = while {
                tunnel: w455 -> [w458]
                tunnel: [w463] -> w456
                tunnel: w457 -> [_]
                tunnel: w454 -> [w461]
                tunnel: [w461] -> w453
                tunnel: [w460] -> w452
                tunnel: w451 -> [w460]
                stop <- w462 continue-if-true
                # "do action"
                n123 = call "BaseSM.change state.vi"("allowed next states"=string[] ["Stand by"], "wait time [ms]"=w458, "i ref in"=w461) -> ("next state"=w463:string, "continue loop"=w462:bool)  [unwired: 13 in, 2 out]
              }
            }
            frame #2 {
              # "exit action"
            }
          }
        }
        frame Default {
          n124 = call "BaseSM.ProcState.vi"("i ref in"=w470, "state timeout [ms]"=w466, "state"=w465, "error in (no error)"=w468) -> ("i ref out"=w469:refnum<vi>, "next state"=w464:string, "error out"=w467:errorcluster)  [unwired: 13 in]
        }
      }
    }
    frame True {
      n125 = call "CoreLib.my to LV error.vi"("ErrorTypes"=CoreDefs.error_type."invalid reference") -> ("myErrorCluster"=w472:errorcluster)  [unwired: 17 in, 1 out]
    }
  }
  "i ref out" <- w8
  "next state" <- w6
  "error out" <- w3
